vi "ClearClassMutationHistory.vi"() -> ()   [LabVIEW 2020]
uses:
  <vilib>/Utility/EditLVLibs/Edit LVLibs.lvlib
panel:
  out "Path":path
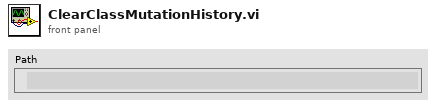
[diagram p1: front panel]
types:
  T1 = typedef "Edit LVLibs.lvlib/Mutation History.ctl" = T2[]
  T2 = typedef "Edit LVLibs.lvlib/Mutation Record.ctl" = cluster{"Library Version":T3, "Old Name Index":u8, "Class Default Data":variant, "Cluster Order Map":u32[], "Parent Name":string, "Parent Path":path, "LabVIEW Version":u32, "User Comments":string, "Mutation Flags":u8, "Parent Old Name Index":u8, "Parent Levels Added":u16, "Parent Levels Removed":u16}
  T3 = typedef "Edit LVLibs.lvlib/LibVersion.ctl" = cluster{"Major":u16, "Minor":u16, "Fix":u16, "Build":u16}
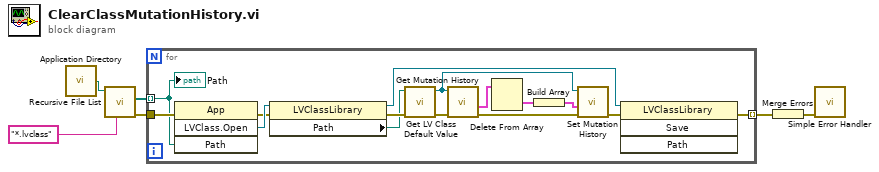
[diagram p0: block diagram]
diagram:
  n1 = call <vilib>:"Application Directory.vi"() -> ("Application Directory"=w6:path)
  n2 = call <vilib>:"Recursive File List.vi"("pattern"="*.lvclass", "Folder Path"=w6) -> ("error out"=w4:errorcluster, "All Files in Dir"=w3:path[])  [unwired: 5 in, 3 out]
  n3 = for {
    tunnel: w4 -> [w17]
    tunnel: w3 -> [w12] mode=indexing
    tunnel: [w9] -> w2 mode=indexing
    n4 = invoke class="App" method="LVClass.Open"(error in=w17, "Path"=w12) -> (error out=w15:errorcluster, "LVClass.Open"=w16:refnum<vi>)  [unwired: 2 in, 2 out]
    n5 = property class="LVClassLibrary"(reference=w16, error in=w15) -> (reference out=w10:refnum<vi>, error out=w14:errorcluster, "Path"=w13:path)
    n6 = call <vilib>:"Get LV Class Default Value.vi"("error in (no error)"=w14, "class path"=w13) -> ("error out"=w21:errorcluster, "object"=w18:refnum<class>)  [unwired: 8 in]
    n7 = call <vilib>:"Get Mutation History.vi"("error in"=w21, "Input object"=w18) -> ("error out"=w19:errorcluster, "Mutation History"=w20:T1)  [unwired: 6 in]
    n8 = Delete From Array(array=w20) -> (deleted portion=w8:T2)  [unwired: 2 in, 1 out]
    n9 = Build Array(w8) -> (w7:T2[])
    n10 = call <vilib>:"Set Mutation History.vi"("error in"=w19, "Mutation History"=w7, "Input object"=w18) -> ("error out"=w11:errorcluster)  [unwired: 8 in]
    n11 = invoke class="LVClassLibrary" method="Save"(reference=w10, error in=w11) -> (error out=w9:errorcluster)  [unwired: 2 in, 3 out]
    "Path" <- w12
  }
  n12 = Merge Errors(w2) -> (w1:errorcluster)
  n13 = call <vilib>:"Simple Error Handler.vi"("error in (no error)"=w1) -> ()  [unwired: 4 in, 5 out]
